vi "ShoulderExecute.vi"(8 "error in (no error)":errorcluster) -> (0 "error out":errorcluster)   [LabVIEW 2023]
doc: "Arm Execute for 2024 robot"
uses:
  <vilib>/Rock Robotics/WPI/ThirdParty/JAS_Junk/TrajLib/Timer_New.vi
  <vilib>/Utility/semaphor.llb/Obtain Semaphore Reference.vi
  <vilib>/Rock Robotics/WPI/ThirdParty/JAS_Junk/TrajLib/Timer_Reset.vi
  <vilib>/Rock Robotics/WPI/ThirdParty/JAS_Junk/TrajLib/Timer_Start.vi
  <vilib>/Rock Robotics/WPI/ThirdParty/JAS_Junk/TrajLib/Timer_HasPeriodPassedOnce.vi
  <vilib>/Rock Robotics/WPI/ThirdParty/JAS_Junk/TrajLib/Timer_Stop.vi
  <vilib>/Rock Robotics/WPI/ThirdParty/JAS_Junk/TrajLib/Trajectory_Library.lvlib
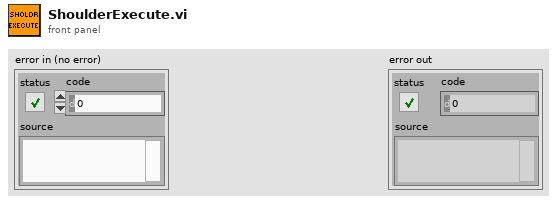
[diagram p1: front panel]
types:
  T1 = typedef "WPI_MotorControlDeviceRef.ctl" = cluster{"DeviceStatus":errorcluster, "Type":T2, "PWM":cluster{"PWM Channel":T3, "DeadBand":T4}, "CAN":cluster{"Device Number":u8, "SetOutput VI Ref":variant, "GetOutput VI Ref":variant, "Enable VI Ref":variant, "Disable VI Ref":variant, "Data":variant}, "Invert":bool, "DIO PWM":cluster{"PWM \"Enable\" Channel":T3, "DIOChannel":T5, "PWM Rate":dbl}}
  T2 = typedef "WPI_MotorControlType.ctl" = enum16{"PWM", "CAN", "DIO PWM"}
  T3 = typedef "FPGA_DIOPWMChannel.ctl" = enum8{"PWM 0", "PWM 1", "PWM 2", "PWM 3", "PWM 4", "PWM 5", "PWM 6", "PWM 7", "PWM 8", "PWM 9", "PWM MXP 0", "PWM MXP 1", "PWM MXP 2", "PWM MXP 3", "PWM MXP 4", "PWM MXP 5", "PWM MXP 6", "PWM MXP 7", "PWM MXP 8", "PWM MXP 9", "Invalid"}
  T4 = typedef "WPI_PWMDeadband.ctl" = cluster{"Name":string, "maxPositivePwm":i32, "minPositivePwm":i32, "centerPwm":i32, "maxNegativePwm":i32, "minNegativePwm":i32, "angularRange":u16}
  T5 = typedef "FPGA_DIOChannel.ctl" = enum8{"DIO 0", "DIO 1", "DIO 2", "DIO 3", "DIO 4", "DIO 5", "DIO 6", "DIO 7", "DIO 8", "DIO 9", "DIO MXP 0", "DIO MXP 1", "DIO MXP 2", "DIO MXP 3", "DIO MXP 4", "DIO MXP 5", "DIO MXP 6", "DIO MXP 7", "DIO MXP 8", "DIO MXP 9", "DIO MXP 10", "DIO MXP 11", "DIO MXP 12", "DIO MXP 13", "DIO MXP 14", "DIO MXP 15", "SPI Port CS1", "SPI Port CS2", "SPI Port CS3", "SPI Port MISO", "SPI Port MOSI", "Invalid"}
  T6 = typedef "WPI_SwitchDevRef.ctl" = cluster{"DevStatus":errorcluster, "DIO Channel":T5, "CntIndex":T7, "Normally Closed":bool}
  T7 = typedef "FPGA_CounterCtrSystemIndex.ctl" = enum8{"Ctr 0", "Ctr 1", "Ctr 2", "Ctr 3", "Ctr 4", "Ctr 5", "Ctr 6", "Ctr 7", "Invalid"}
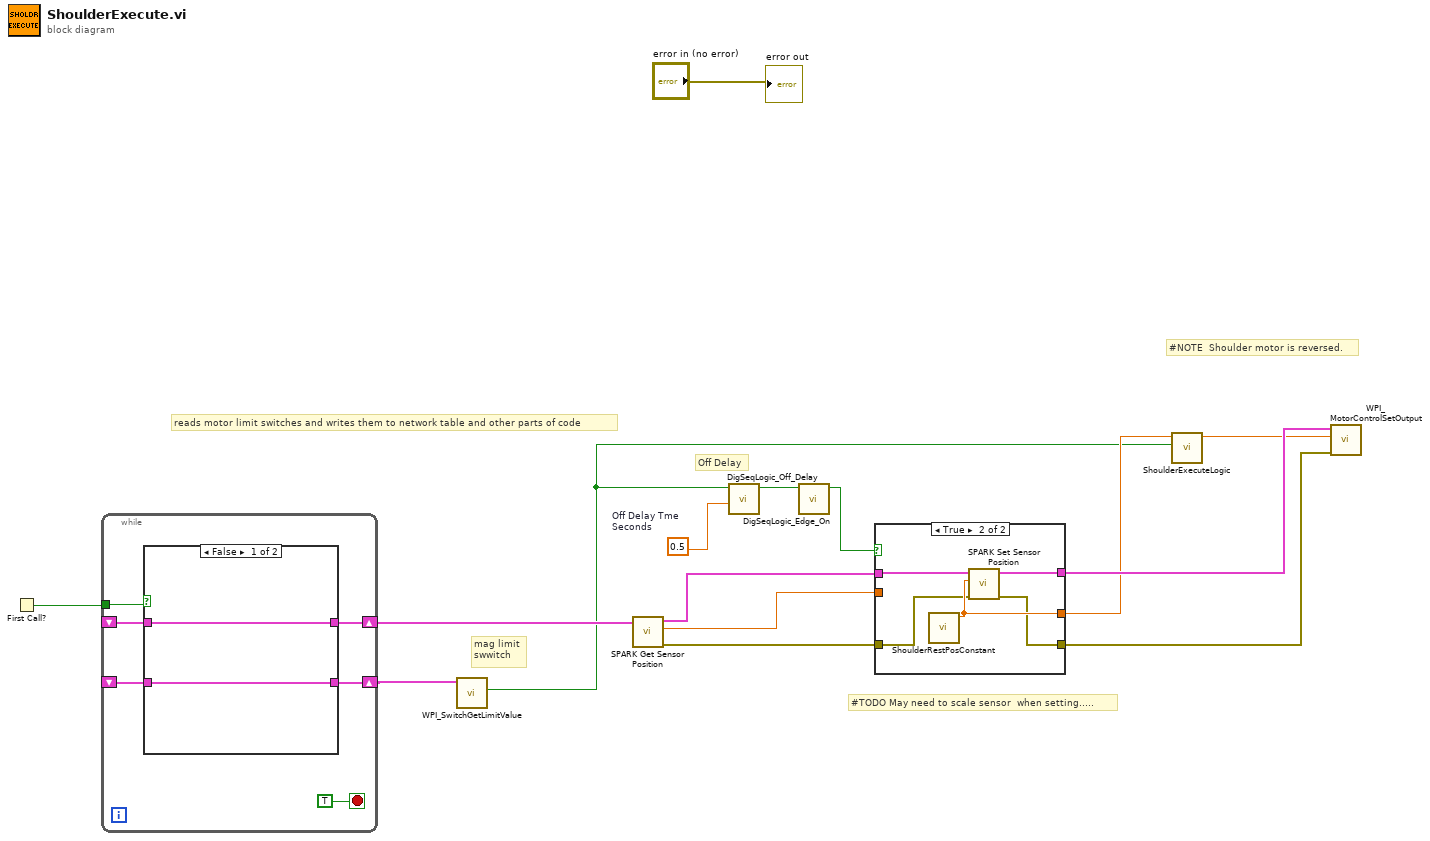
[diagram p0: block diagram]
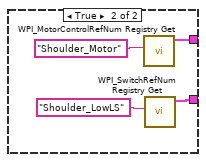
[diagram p2: hidden frame]
diagram:
  w9 = 0.5  # Off Delay Tme Seconds
  # "#NOTE  Shoulder motor is reversed."
  # "#TODO May need to scale sensor  when setting....."
  # "Off Delay"
  # "mag limit\nswwitch"
  # "reads motor limit switches and writes them to network table and other parts of code"
  n1 = First Call?() -> (First Call?: T/F=w12:bool)
  n2 = while {
    tunnel: w12 -> [w20]
    shift-right: [w21] -> w10
    shift-left: _ -> [w18]
    shift-right: [w17] -> w3
    shift-left: _ -> [w16]
    stop <- TRUE stop-if-true
    n3 = case shown="False" w20 {
      tunnel: [w23 w27] -> w21
      tunnel: w18 -> [w23 _]
      tunnel: [w22 w25] -> w17
      tunnel: w16 -> [w22 _]
      frame False {
      }
      frame True {
        n4 = call <vilib>:"WPI_MotorControlRefNum Registry Get.vi"("refnum name"="Shoulder_Motor") -> ("MotorControlDevRef"=w27:T1)  [unwired: 9 in, 1 out]
        n5 = call <vilib>:"WPI_SwitchRefNum Registry Get.vi"("refnum name"="Shoulder_LowLS") -> ("SwitchDevRef"=w25:T6)  [unwired: 9 in, 1 out]
      }
    }
  }
  n6 = call <vilib>:"WPI_SwitchGetLimitValue.vi"("SwitchDevRef"=w3) -> ("Switch Pressed"=w2:bool)  [unwired: 8 in, 2 out]
  n7 = call <vilib>:"SPARK Get Sensor Position.vi"("MotorControlDevRef in"=w10) -> ("error out"=w5:errorcluster, "Sensor Position"=w6:dbl, "MotorControlDevRef out"=w14:T1)  [unwired: 7 in, 1 out]
  n8 = call <vilib>:"DigSeqLogic_Off_Delay.vi"("Delay"=w9, "Input"=w2) -> ("Output"=w8:bool)  [unwired: 8 in, 1 out]
  n9 = call <vilib>:"DigSeqLogic_Edge_On.vi"("Input"=w8) -> ("On Edge"=w13:bool)  [unwired: 10 in]
  n10 = case shown="True" w13 {
    tunnel: [w30 w35] -> w11
    tunnel: w14 -> [w30 w34]
    tunnel: [w29 w33] -> w7
    tunnel: w6 -> [w29 _]
    tunnel: w5 -> [w28 w32]
    tunnel: [w28 w31] -> w4
    frame False {
    }
    frame True {
      n11 = call "ShoulderRestPosConstant.vi"() -> ("RestPosition"=w33:dbl)  [unwired: 11 in]
      n12 = call <vilib>:"SPARK Set Sensor Position.vi"("error in"=w32, "Position"=w33, "MotorControlDeviceRef"=w34) -> ("error out"=w31:errorcluster, "MotorControlDeviceRef"=w35:T1)  [unwired: 7 in]
    }
  }
  n13 = call "ShoulderExecuteLogic.vi"("LowLimitSwitch"=w2, "PositionDeg"=w7) -> ("MotorDemand"=w1:dbl)  [unwired: 8 in, 1 out]
  n14 = call <vilib>:"WPI_MotorControlSetOutput.vi"("error in (no error)"=w4, "Output"=w1, "MotorControlDevRef"=w11) -> ()  [unwired: 6 in, 3 out]
  "error out" <- "error in (no error)"
